vi "dfd_Get Gain Type.vi"(9 "sum iwl":i16, 10 "gain value":dbl, 11 "gain wl":i16) -> (1 "output iwl":i32, 3 "gain type":T1(ring))   [LabVIEW 2017, in "NI_DigFilterLicensed.lvlib"]
uses:
  <vilib>/addons/Digital Filter Design/NI_DigFilterLicensed.lvlib
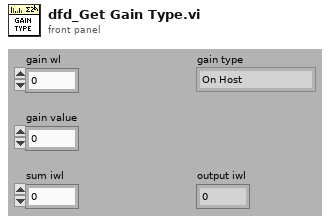
[diagram p1: front panel]
types:
  T1 = enum16{"On Host", "Power of 2", "Non-power of 2"}
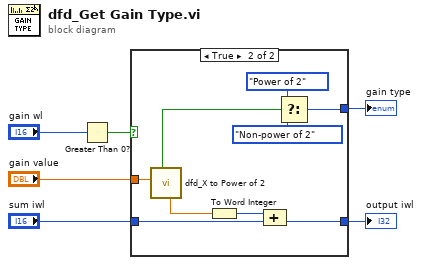
[diagram p0: block diagram]
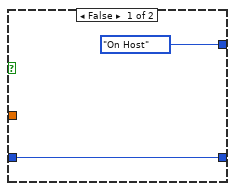
[diagram p2: hidden frame]
diagram:
  n1 = Greater Than 0?(x="gain wl") -> (x > 0?=w2:bool)
  n2 = case shown="True" w2 {
    tunnel: [w8 w13] -> w6
    tunnel: "sum iwl" -> [w8 w17]
    tunnel: "gain value" -> [_ w16]
    tunnel: [T1."On Host" ("gain type") w11] -> w1
    frame False {
    }
    frame True {
      n3 = call <vilib>:"dfd_X to Power of 2.vi"("x"=w16) -> ("n"=w14:dbl, "is 2^n?"=w12:bool)  [unwired: 9 out]
      n4 = To Word Integer(number=w14) -> (16bit integer=w15:i16)
      n5 = Compound Arithmetic op=ADD(w15, w17) -> (w13:i16)
      n6 = Select(t=T1."Power of 2" ("gain type"), s=w12, f=T1."Non-power of 2" ("gain type")) -> (s? t:f=w11:T1)
    }
  }
  "output iwl" <- w6
  "gain type" <- w1
